vi "Tenney_Read_Viasala_Humidity.vi"(0 "Message Queues out":T2, 1 "Enable Averaging":bool, 7 "Enable Arrays":bool, 9 "Loop Count Ref":refnum<vi>, 11 "error in":errorcluster, 13 "Connect Viasala Ref":refnum<vi>, 14 "Viasala Array":refnum<vi>) -> (15 "error out":errorcluster)   [LabVIEW 2023]
uses:
  Message Queue/All Message Queues.ctl
  Message Queue/Message Cluster.ctl
  Drivers/Viasala Indigo 520/Type Definitions/Viasala Indigo 520 Data.ctl
  Message Queue/Enqueue Message (Single).vi
  FVIR and LDO/support/Message Queue/Enqueue Message (Single).vi
  <vilib>/NI/Modbus Library/API/Master/Modbus Master.lvclass
  Message Queue/Tenney Message Queue.lvlib
  FVIR and LDO/support/Message Queue/Message Queue.lvlib
panel:
  out "String":string
  out "Connect Viasala Counter":dbl
  out "Viasala Data Output":T1
  out "appended array":string[](array[string])
  out "Loop Count":i32
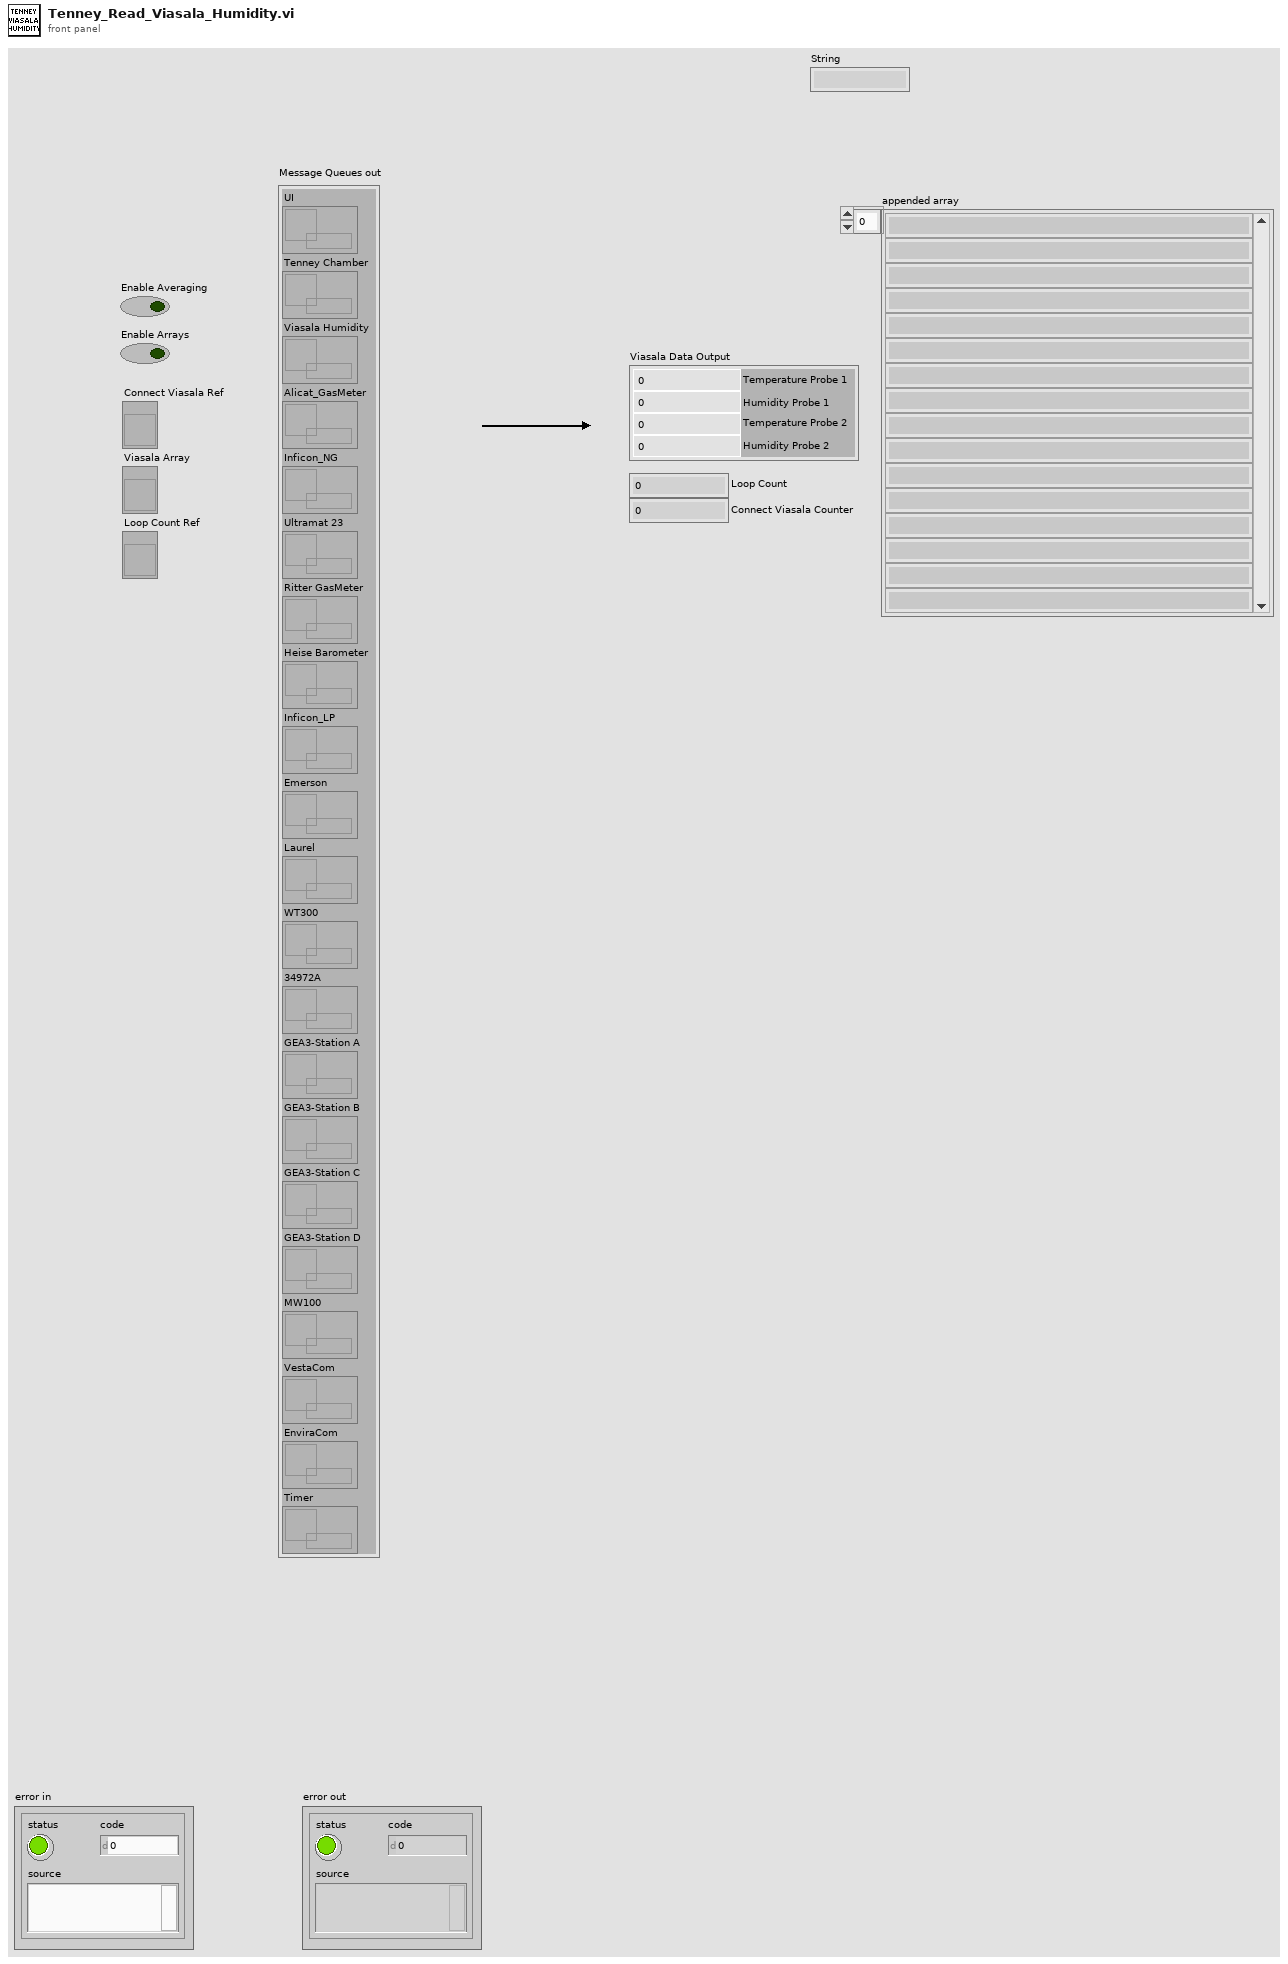
[diagram p1: front panel]
types:
  T1 = typedef "Viasala Indigo 520 Data.ctl" = cluster{"Temperature Probe 1":dbl, "Humidity Probe 1":dbl, "Temperature Probe 2":dbl, "Humidity Probe 2":dbl}
  T2 = typedef "Tenney Message Queue.lvlib/All Message Queues.ctl" = cluster{"UI":refnum<queue>, "Tenney Chamber":refnum<queue>, "Viasala Humidity":refnum<queue>, "Alicat_GasMeter":refnum<queue>, "Inficon_NG":refnum<queue>, "Ultramat 23":refnum<queue>, "Ritter GasMeter":refnum<queue>, "Heise Barometer":refnum<queue>, "Inficon_LP":refnum<queue>, "Emerson":refnum<queue>, "Laurel":refnum<queue>, "WT300":refnum<queue>, "34972A":refnum<queue>, "GEA3-Station A":refnum<queue>, "GEA3-Station B":refnum<queue>, "GEA3-Station C":refnum<queue>, "GEA3-Station D":refnum<queue>, "MW100":refnum<queue>, "VestaCom":refnum<queue>, "EnviraCom":refnum<queue>, "Timer":refnum<queue>}
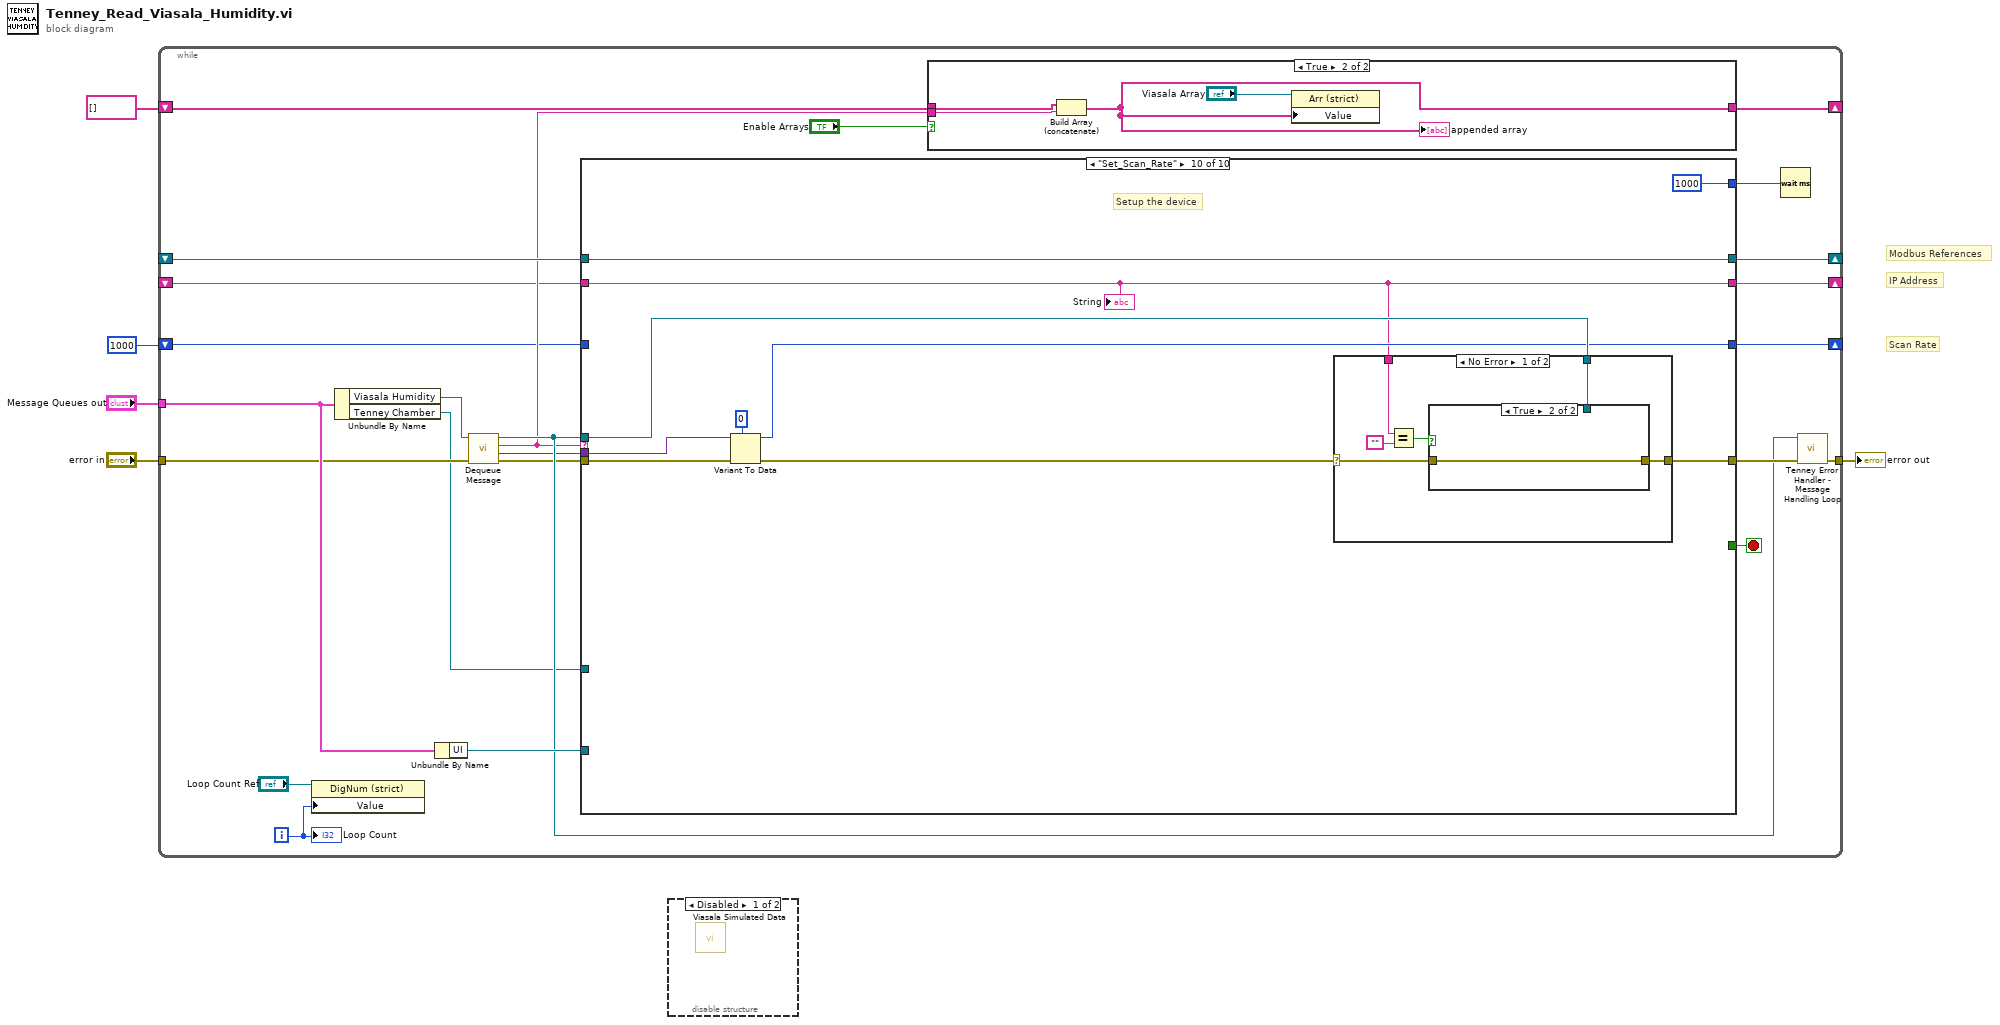
[diagram p0: block diagram]
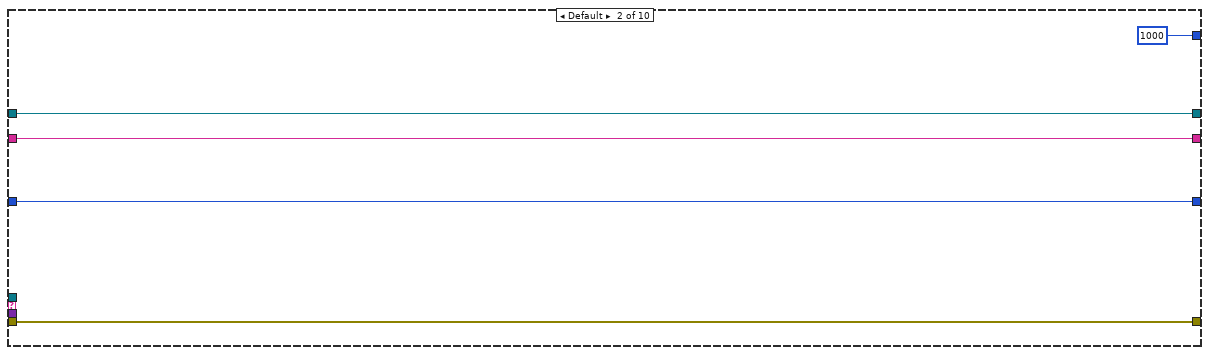
[diagram p5: hidden frame]
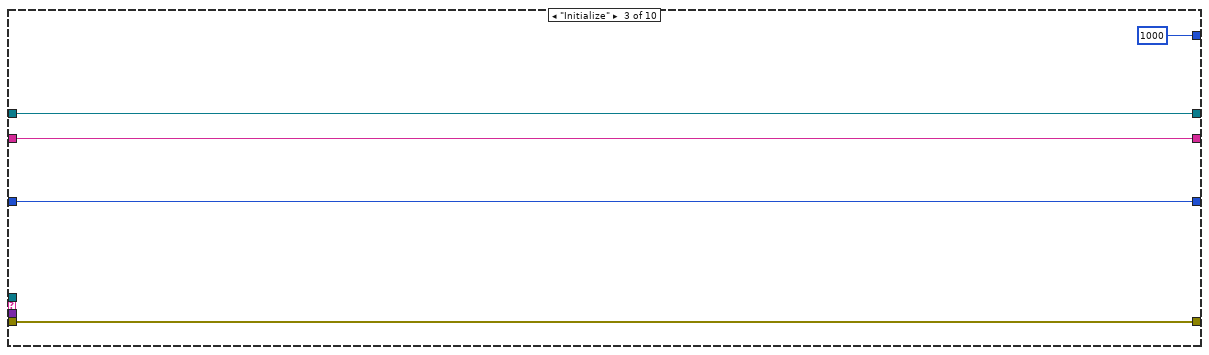
[diagram p6: hidden frame]
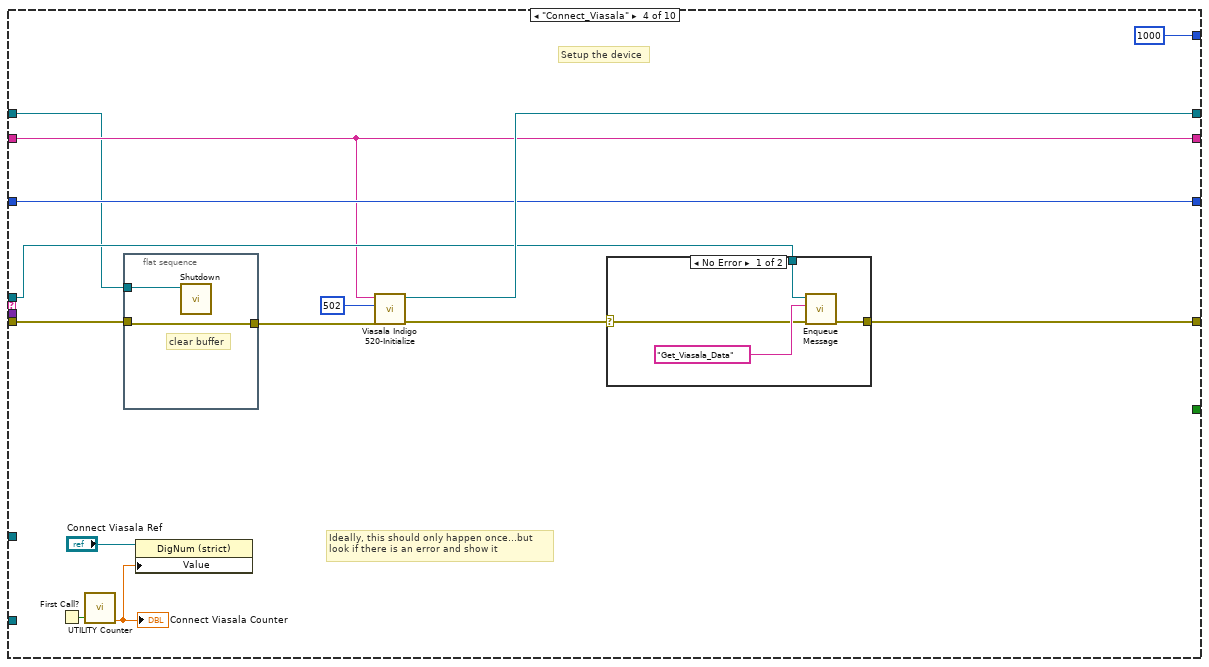
[diagram p7: hidden frame]
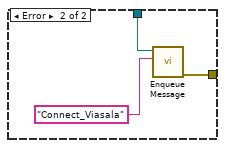
[diagram p8: hidden frame]
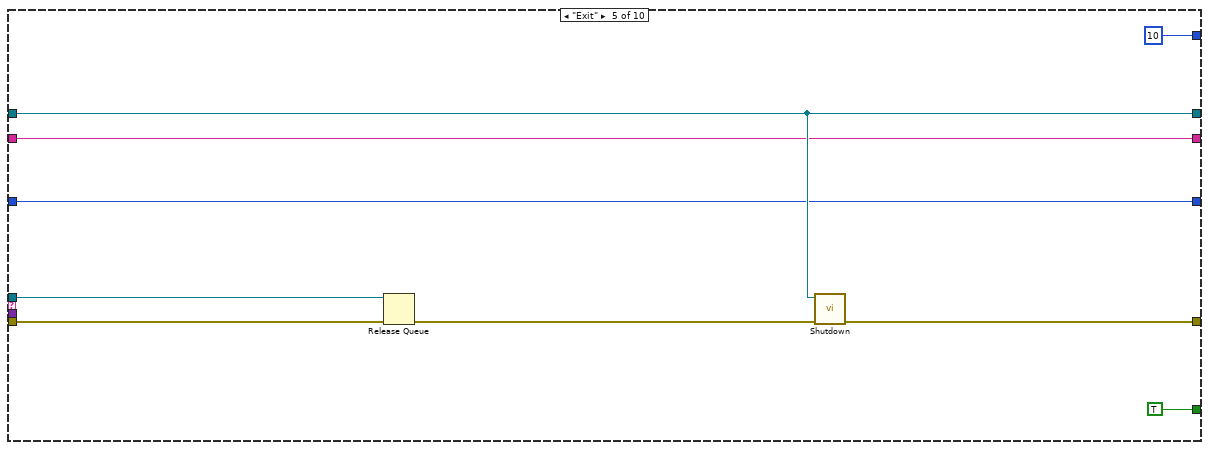
[diagram p9: hidden frame]
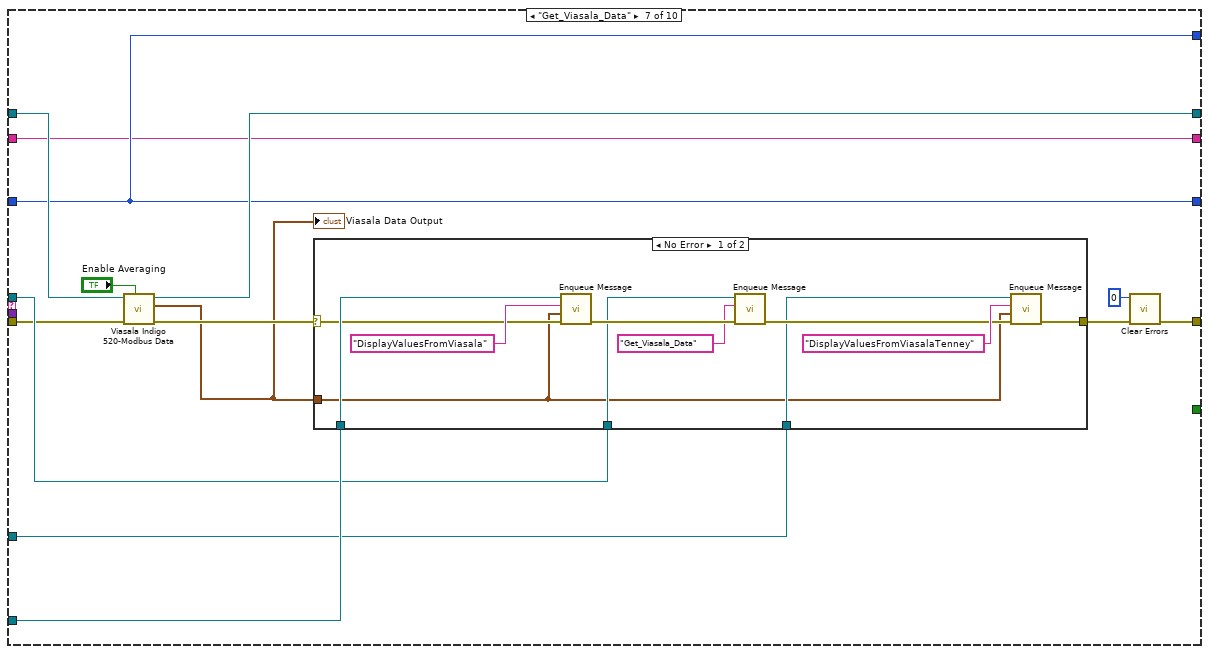
[diagram p11: hidden frame]
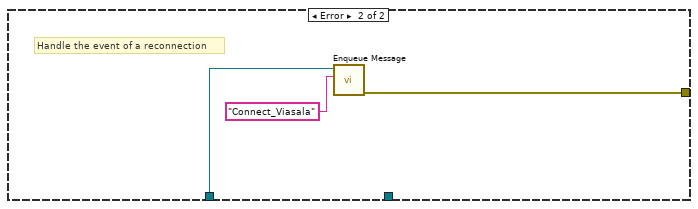
[diagram p12: hidden frame]
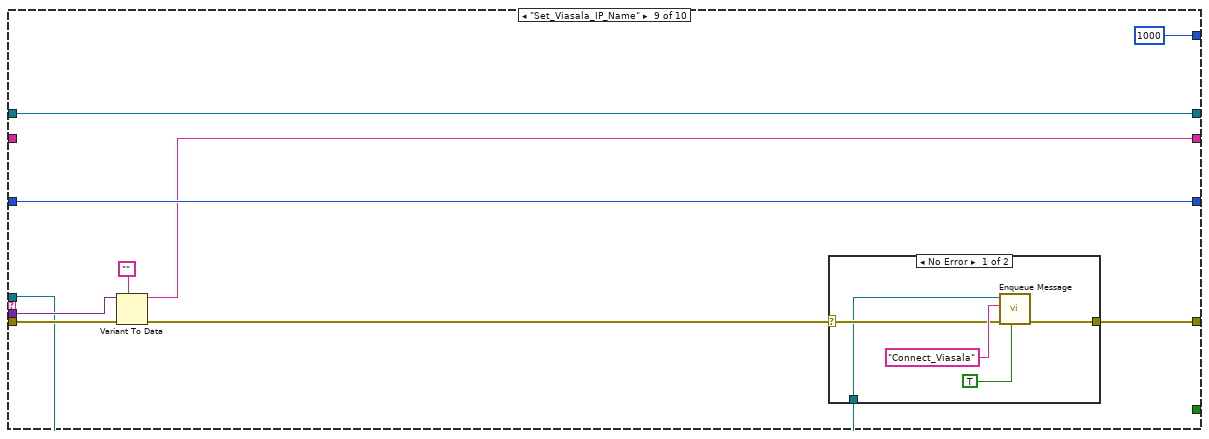
[diagram p14: hidden frame]
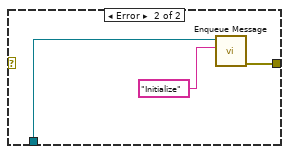
[diagram p15: hidden frame]
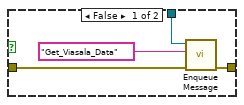
[diagram p16: hidden frame]
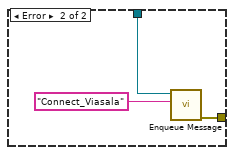
[diagram p17: hidden frame]
diagram:
  # "Scan Rate"
  # "Modbus References"
  # "IP Address"
  n1 = while {
    tunnel: "Message Queues out" -> [w26]
    tunnel: "error in" -> [w22]
    tunnel: [w28] -> w4
    shift-right: [w19] -> _
    shift-left: _ -> [w18]
    shift-right: [w15] -> _
    shift-left: string[] [] -> [w16]
    shift-right: [w10] -> _
    shift-left: u32 1000 ("millisecond multiple") -> [w9]
    shift-right: [w7] -> _
    shift-left: _ -> [w6]
    i -> [w11]
    stop <- w29 stop-if-true
    n2 = property class="DigNum (strict)"(reference="Loop Count Ref", "Value"=w11) -> ()  [unwired: 1 in, 2 out]
    n3 = Unbundle By Name(w26) -> ("Viasala Humidity"=w24:refnum<queue>, "Tenney Chamber"=w13:refnum<queue>)
    n4 = Unbundle By Name(w26) -> ("UI"=w25:refnum<queue>)
    n5 = call "Dequeue Message.vi"("error in (no error)"=w22, "Message Queue"=w24) -> ("error out"=w21:errorcluster, "Message Data"=w20:variant, "Message"=w14:string, "dup Message Queue"=w23:refnum<queue>)  [unwired: 6 in]
    n6 = case shown="\"Set_Scan_Rate\"" w14 {
      tunnel: w21 -> [w37 w41 w45 w51 w74 w83 w96 w115 w122 w142]
      tunnel: [w37 w41 w45 w49 w78 w83 w87 w115 w119 w136] -> w27
      tunnel: [_ _ _ _ TRUE _ _ _ _ _] -> w29
      tunnel: w23 -> [_ _ _ w58 w75 _ w97 _ w118 w139]
      tunnel: w25 -> [_ _ _ _ _ _ w98 _ _ _]
      tunnel: w20 -> [_ _ _ _ _ _ _ _ w120 w141]
      tunnel: [w38 w43 w48 w61 w77 w84 w94 w116 w126 w137] -> w19
      tunnel: w18 -> [w38 w43 w48 w52 w77 w84 w95 w116 w126 w137]
      tunnel: [w36 u32 1000 ("millisecond multiple") u32 1000 ("millisecond multiple") u32 1000 ("millisecond multiple") u32 10 ("millisecond multiple") w82 w90 w114 u32 1000 ("millisecond multiple") u32 1000 ("millisecond multiple")] -> w17
      tunnel: w13 -> [_ _ _ _ _ _ w91 _ _ _]
      tunnel: [w36 w40 w46 w59 w73 w82 w90 w114 w124 w138] -> w10
      tunnel: w9 -> [w36 w40 w46 w59 w73 w82 w90 w114 w124 _]
      tunnel: [w35 w39 w44 w54 w72 w81 w86 w113 w117 w135] -> w7
      tunnel: w6 -> [w35 w39 w44 w54 w72 w81 w86 w113 _ w135]
      frame "---------- Setup ----------" {
      }
      frame Default {
      }
      frame "Initialize" {
      }
      frame "Connect_Viasala" {
        # "Ideally, this should only happen once...but\nlook if there is an error and show it"
        # "Setup the device"
        n7 = First Call?() -> (First Call?: T/F=w55:bool)
        n8 = call "UTILITY Counter.vi"("Reset"=w55) -> ("Count"=w57:dbl)  [unwired: 10 in]
        "Connect Viasala Counter" <- w57
        n9 = flat-sequence {
          tunnel: w52 -> [w64]
          tunnel: w51 -> [w63]
          tunnel: [w63] -> w50
          frame #0 {
            # "clear buffer"
            n10 = call-dynamic "Shutdown.vi"("Modbus master in"=w64) -> ()  [unwired: 10 in, 1 out]
          }
        }
        n11 = property class="DigNum (strict)"(reference="Connect Viasala Ref", "Value"=w57) -> ()  [unwired: 1 in, 2 out]
        n12 = call "Viasala Indigo 520-Initialize.vi"("error in (no error)"=w50, "Remote Port"=u16 502, "IP Address"=w54) -> ("error out"=w62:errorcluster, "Modbus Master out"=w61:refnum<class "Modbus Master.lvclass">)  [unwired: 7 in]
        n13 = case shown="No Error" w62 {
          selector: w62 -> [w65 _]
          tunnel: w58 -> [w67 w70]
          tunnel: [w66 w71] -> w49
          frame No Error {
            n14 = call-poly "Enqueue Message.vi"("error in (no error)"=w65, "Message"="Get_Viasala_Data", "Message Queue"=w67) -> ("error out"=w66:errorcluster)  [unwired: 7 in, 1 out]
          }
          frame Error {
            n15 = call-poly "Enqueue Message.vi"("Message"="Connect_Viasala", "Message Queue"=w70) -> ("error out"=w71:errorcluster)  [unwired: 8 in, 1 out]
          }
        }
      }
      frame "Exit" {
        n16 = Release Queue(queue=w75, error in (no error)=w74) -> (error out=w79:errorcluster)  [unwired: 1 in, 2 out]
        n17 = call-dynamic "Shutdown.vi"("error in"=w79, "Modbus master in"=w77) -> ("error out"=w78:errorcluster)  [unwired: 9 in]
      }
      frame "---------- Data Collection ----------" {
      }
      frame "Get_Viasala_Data" {
        n18 = call "Viasala Indigo 520-Modbus Data.vi"("Enable Averaging"="Enable Averaging", "error in (no error)"=w96, "Modbus master in"=w95) -> ("error out"=w93:errorcluster, "Viasala Data Output"=w92:T1, "Modbus master out"=w94:refnum<class "Modbus Master.lvclass">)  [unwired: 5 in, 1 out]
        "Viasala Data Output" <- w92
        n19 = case shown="No Error" w93 {
          selector: w93 -> [w107 _]
          tunnel: w98 -> [w108 _]
          tunnel: [w101 w112] -> w88
          tunnel: w97 -> [w105 w110]
          tunnel: w92 -> [w99 _]
          tunnel: w91 -> [w100 _]
          frame No Error {
            n20 = call-poly "Enqueue Message.vi"("error in (no error)"=w107, "Message Data"=w99, "Message"="DisplayValuesFromViasala", "Message Queue"=w108) -> ("error out"=w106:errorcluster)  [unwired: 6 in, 1 out]
            n21 = call-poly "Enqueue Message.vi"("error in (no error)"=w106, "Message"="Get_Viasala_Data", "Message Queue"=w105) -> ("error out"=w102:errorcluster)  [unwired: 7 in, 1 out]
            n22 = call-poly "Enqueue Message.vi"("error in (no error)"=w102, "Message Data"=w99, "Message"="DisplayValuesFromViasalaTenney", "Message Queue"=w100) -> ("error out"=w101:errorcluster)  [unwired: 6 in, 1 out]
          }
          frame Error {
            # "Handle the event of a reconnection"
            n23 = call-poly "Enqueue Message.vi"("Message"="Connect_Viasala", "Message Queue"=w110) -> ("error out"=w112:errorcluster)  [unwired: 8 in, 1 out]
          }
        }
        n24 = call <vilib>:"Clear Errors.vi"("error in (no error)"=w88, "specific error code to clear (0: all)"=0) -> ("error out"=w87:errorcluster)  [unwired: 4 in, 1 out]
      }
      frame "---------- Events ----------" {
      }
      frame "Set_Viasala_IP_Name" {
        n25 = Variant To Data(error in=w122, type="", Variant=w120) -> (data=w117:string, error out=w121:errorcluster)
        n26 = case shown="No Error" w121 {
          selector: w121 -> [w129 _]
          tunnel: [w128 w133] -> w119
          tunnel: w118 -> [w127 w132]
          frame No Error {
            n27 = call-poly "Enqueue Message.vi"("Priority Message? (F)"=TRUE, "error in (no error)"=w129, "Message"="Connect_Viasala", "Message Queue"=w127) -> ("error out"=w128:errorcluster)  [unwired: 6 in, 1 out]
          }
          frame Error {
            n28 = call-poly "Enqueue Message.vi"("Message"="Initialize", "Message Queue"=w132) -> ("error out"=w133:errorcluster)  [unwired: 8 in, 1 out]
          }
        }
      }
      frame "Set_Scan_Rate" {
        # "Setup the device"
        n29 = Variant To Data(error in=w142, type=u32 0, Variant=w141) -> (data=w138:u32, error out=w140:errorcluster)
        n30 = case shown="No Error" w140 {
          selector: w140 -> [w149 _]
          tunnel: [w150 w158] -> w136
          tunnel: w139 -> [w148 w156]
          tunnel: w135 -> [w145 _]
          frame No Error {
            n31 = Equal?(x=w145, y="") -> (x = y?=w147:bool)
            n32 = case shown="True" w147 {
              tunnel: [w154 w155] -> w150
              tunnel: w149 -> [w153 w155]
              tunnel: w148 -> [w152 _]
              frame False {
                n33 = call-poly "Enqueue Message.vi"("error in (no error)"=w153, "Message"="Get_Viasala_Data", "Message Queue"=w152) -> ("error out"=w154:errorcluster)  [unwired: 7 in, 1 out]
              }
              frame True {
              }
            }
          }
          frame Error {
            n34 = call-poly "Enqueue Message.vi"("Message"="Connect_Viasala", "Message Queue"=w156) -> ("error out"=w158:errorcluster)  [unwired: 8 in, 1 out]
          }
        }
        "String" <- w135
      }
    }
    n35 = case shown="True" "Enable Arrays" {
      tunnel: w16 -> [w30 w34]
      tunnel: [w30 w31] -> w15
      tunnel: w14 -> [_ w33]
      frame False {
      }
      frame True {
        n36 = Build Array (concatenate)(w34, w33) -> (w31:string[])
        "appended array" <- w31
        n37 = property class="Arr (strict)"(reference="Viasala Array", "Value"=w31) -> ()  [unwired: 1 in, 2 out]
      }
    }
    n38 = Wait (ms)(milliseconds to wait=w17) -> ()  [unwired: 1 out]
    n39 = call "Tenney Error Handler - Message Handling Loop.vi"("error in (no error)"=w27, "Message Queue"=w23) -> ("dup error in"=w28:errorcluster)  [unwired: 8 in, 1 out]
    "Loop Count" <- w11
  }
  "error out" <- w4
  n40 = disable-structure shown="Disabled" {
    frame Disabled {
      n41 = call "Viasala Simulated Data.vi"() -> ()  [unwired: 10 in, 2 out]
    }
    frame Enabled {
    }
  }
